vi "RT update PID parameters.vi"(2 "error in":errorcluster, 3 "FPGA Parameter cluster":T1={"Output settings"={"Relay Switch Matrix"=0, "Set output"=[0.0, 0.0, 0.0, 0.0], "set output?"=FALSE, "set relay matrix?"=FALSE}, "PID settings"={"PID input channel"=enum."PID Disabled", "PID output channel"=enum."PID Disabled", "PID gains"={"proportional gain"=0.0, "integral gain"=0.0, "derivative gain"=0.0, "filter coefficient"=0.0}, "PID output ranges"={"output high (Inf)"=0.0, "output low (-Inf)"=0.0}, "Setpoint for PID input chn"=0.0, "config PID gain?"=FALSE, "reset PID?"=FALSE, "config PID range?"=FALSE, "config PID input?"=FALSE, "config PID output?"=FALSE, "config PID setpoint?"=FALSE}, "NI9219 Settings"={"9219 Conversion Time"=enum."High Speed", "Input voltage range"=[0, 0, 0, 0], "config 9219 conversion time?"=FALSE, "config 9219 input range?"=FALSE}, "REQUEST_ID"=0} {"REQUEST_ID" format="%x"; "NI9219 Settings"."Input voltage range" items=["+/- 60V", "+/- 15V", "+/- 4V", "+/- 1V", "+/- 125mV"]}, 4 "FPGA VI ref in":refnum<k20>) -> (0 "error out":errorcluster, 1 "FPGA VI Reference Out":refnum<k20>)   [LabVIEW 2016]
uses:
  Type Def Ctrls/RT ctrls/FPGA parameter cluster.ctl
  Type Def Ctrls/FPGA ctrls/NI9219VoltageRange.ctl
  <vilib>/Utility/error.llb/Error Cluster From Error Code.vi
  <vilib>/rvi/errors/niLvFpgaAdjustHostInterfaceError.vi
  <vilib>/rvi/interface/nirviReadWriteControl/nirviReadWriteControl.xnode
  <vilib>/rvi/interface/Simulation/niFpgaSimulationCallBeginRW.vi
  NiFpgaLv.dll
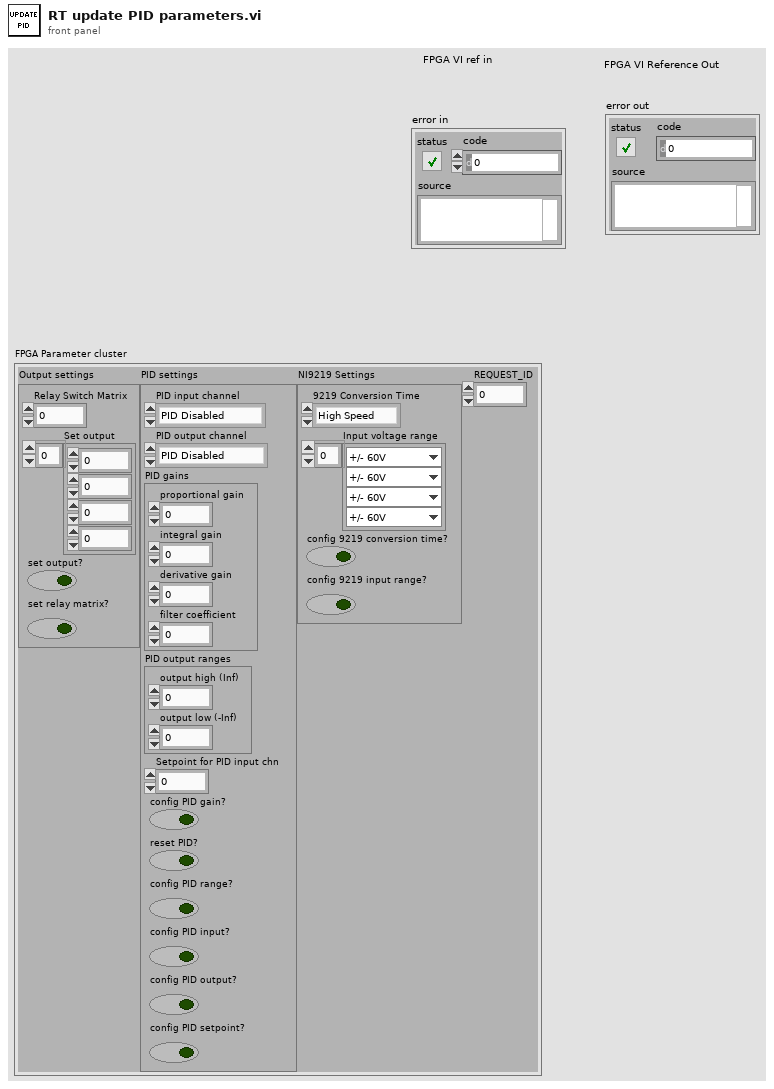
[diagram p1: front panel]
types:
  T1 = typedef "FPGA parameter cluster.ctl" = cluster{"Output settings":cluster{"Relay Switch Matrix":u32, "Set output":sgl[], "set output?":bool, "set relay matrix?":bool}, "PID settings":cluster{"PID input channel":enum16{"Output Channel 0", "Output Channel 1", "Output Channel 2", "Output Channel 3", "PID Disabled"}, "PID output channel":enum16{"Output Channel 0", "Output Channel 1", "Output Channel 2", "Output Channel 3", "PID Disabled"}, "PID gains":cluster{"proportional gain":sgl, "integral gain":sgl, "derivative gain":sgl, "filter coefficient":sgl}, "PID output ranges":cluster{"output high (Inf)":sgl, "output low (-Inf)":sgl}, "Setpoint for PID input chn":sgl, "config PID gain?":bool, "reset PID?":bool, "config PID range?":bool, "config PID input?":bool, "config PID output?":bool, "config PID setpoint?":bool}, "NI9219 Settings":cluster{"9219 Conversion Time":enum8{"High Speed", "Best 60 Hz Rejection", "Best 50 Hz Rejection", "High Resolution"}, "Input voltage range":T2[], "config 9219 conversion time?":bool, "config 9219 input range?":bool}, "REQUEST_ID":u64}
  T2 = typedef "NI9219VoltageRange.ctl" = u8
  T3 = enum16{"Output Channel 0", "Output Channel 1", "Output Channel 2", "Output Channel 3", "PID Disabled"}
  T4 = cluster{"proportional gain":sgl, "integral gain":sgl, "derivative gain":sgl, "filter coefficient":sgl}
  T5 = cluster{"output high (Inf)":sgl, "output low (-Inf)":sgl}
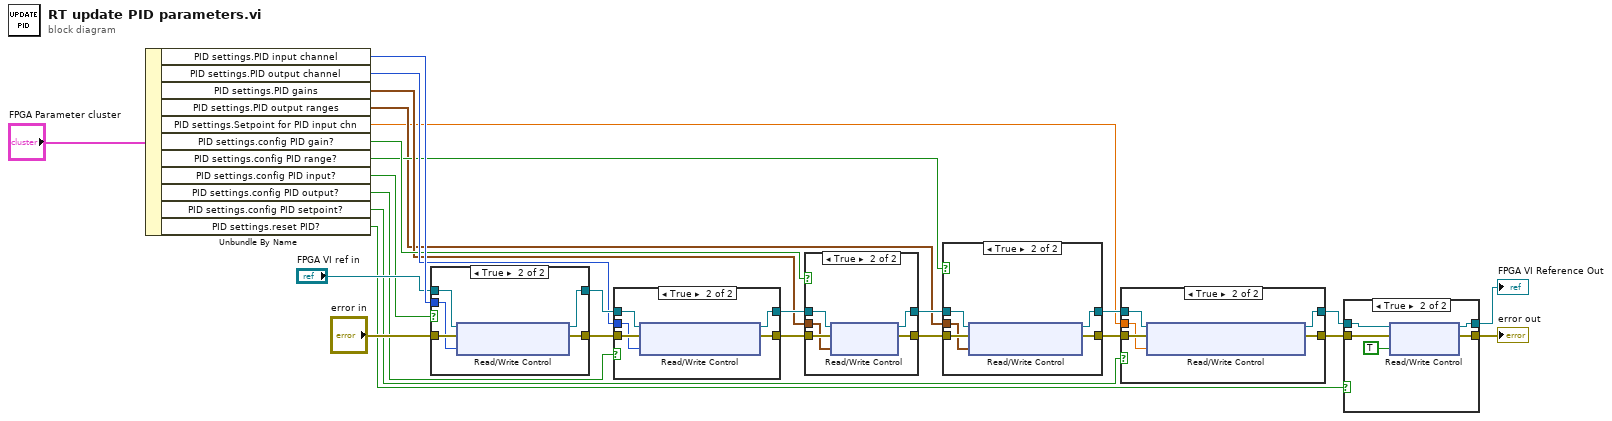
[diagram p0: block diagram]
diagram:
  n1 = Unbundle By Name("FPGA Parameter cluster") -> ("PID settings.PID input channel"=w26:T3, "PID settings.PID output channel"=w12:T3, "PID settings.PID gains"=w10:T4, "PID settings.PID output ranges"=w8:T5, "PID settings.Setpoint for PID input chn"=w6:sgl, "PID settings.config PID gain?"=w11:bool, "PID settings.config PID range?"=w9:bool, "PID settings.config PID input?"=w22:bool, "PID settings.config PID output?"=w13:bool, "PID settings.config PID setpoint?"=w7:bool, "PID settings.reset PID?"=w3:bool)
  n2 = case shown="True" w22 {
    tunnel: "FPGA VI ref in" -> [w28 w33]
    tunnel: [w28 w32] -> w21
    tunnel: "error in" -> [w27 w31]
    tunnel: [w27 w30] -> w20
    tunnel: w26 -> [_ w29]
    frame False {
    }
    frame True {
      n3 = xnode "Read/Write Control"("FPGA VI Reference In"=w33, "error in"=w31, "PID input channel"=w29) -> ("FPGA VI Reference Out"=w32:refnum<k20>, "error out"=w30:errorcluster)
    }
  }
  n4 = case shown="True" w13 {
    tunnel: w21 -> [w35 w40]
    tunnel: w20 -> [w34 w39]
    tunnel: [w35 w38] -> w19
    tunnel: [w34 w37] -> w18
    tunnel: w12 -> [_ w36]
    frame False {
    }
    frame True {
      n5 = xnode "Read/Write Control"("FPGA VI Reference In"=w40, "error in"=w39, "PID output channel"=w36) -> ("FPGA VI Reference Out"=w38:refnum<k20>, "error out"=w37:errorcluster)
    }
  }
  n6 = case shown="True" w11 {
    tunnel: w19 -> [w42 w47]
    tunnel: w18 -> [w41 w46]
    tunnel: [w42 w45] -> w17
    tunnel: [w41 w44] -> w16
    tunnel: w10 -> [_ w43]
    frame False {
    }
    frame True {
      n7 = xnode "Read/Write Control"("FPGA VI Reference In"=w47, "error in"=w46, "PID gains"=w43) -> ("FPGA VI Reference Out"=w45:refnum<k20>, "error out"=w44:errorcluster)
    }
  }
  n8 = case shown="True" w9 {
    tunnel: w17 -> [w49 w54]
    tunnel: w16 -> [w48 w53]
    tunnel: [w49 w52] -> w15
    tunnel: [w48 w51] -> w14
    tunnel: w8 -> [_ w50]
    frame False {
    }
    frame True {
      n9 = xnode "Read/Write Control"("FPGA VI Reference In"=w54, "error in"=w53, "PID output ranges"=w50) -> ("FPGA VI Reference Out"=w52:refnum<k20>, "error out"=w51:errorcluster)
    }
  }
  n10 = case shown="True" w7 {
    tunnel: w15 -> [w56 w61]
    tunnel: w14 -> [w55 w60]
    tunnel: w6 -> [_ w59]
    tunnel: [w56 w58] -> w5
    tunnel: [w55 w57] -> w4
    frame False {
    }
    frame True {
      n11 = xnode "Read/Write Control"("FPGA VI Reference In"=w61, "error in"=w60, "Setpoint for  PID input chn"=w59) -> ("FPGA VI Reference Out"=w58:refnum<k20>, "error out"=w57:errorcluster)
    }
  }
  n12 = case shown="True" w3 {
    tunnel: w5 -> [w63 w68]
    tunnel: w4 -> [w62 w67]
    tunnel: [w63 w65] -> w2
    tunnel: [w62 w64] -> w1
    frame False {
    }
    frame True {
      n13 = xnode "Read/Write Control"("FPGA VI Reference In"=w68, "error in"=w67, "reset PID?"=TRUE) -> ("FPGA VI Reference Out"=w65:refnum<k20>, "error out"=w64:errorcluster)
    }
  }
  "FPGA VI Reference Out" <- w2
  "error out" <- w1
